vi "Destroy.vi"(8 "error in (no error)":errorcluster, 11 "Control In":refnum<class "Control.lvclass">) -> (0 "error out":errorcluster, 3 "Control Out":refnum<class "Control.lvclass">)   [LabVIEW 2015, in "Front Panel Publisher.lvlib" / "Control.lvclass"]
uses:
  Control.lvclass
  Object_class/Object.lvclass
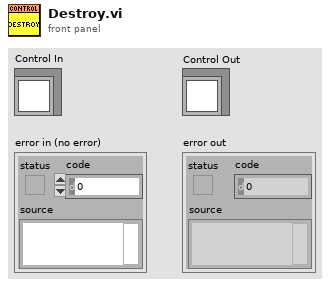
[diagram p1: front panel]
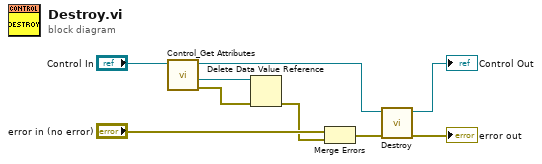
[diagram p0: block diagram]
diagram:
  n1 = call "Control_Get Attributes.vi"("Control In"="Control In") -> ("error out"=w8:errorcluster, "DataRef"=w7:refnum<data-value>, "Control Out"=w2:refnum<class "Control.lvclass">)  [unwired: 7 in, 1 out]
  n2 = Delete Data Value Reference(data value reference=w7, error in=w8) -> (error out=w5:errorcluster)  [unwired: 1 out]
  n3 = Merge Errors("error in (no error)", w5) -> (w4:errorcluster)
  n4 = call-parent "Destroy.vi"("error in (no error)"=w4, "Object In"=w2) -> ("error out"=→"error out":errorcluster, "Object Out"=→"Control Out":refnum<class "Control.lvclass">)  [unwired: 8 in]
